vi "nanostage-reset.vi"(3 "error in":errorcluster, 4 "reset stage":bool, 5 "All conn. axes":string[](array[string])) -> (0 "error out":errorcluster, 2 "Error Description":string)   [LabVIEW 2017]
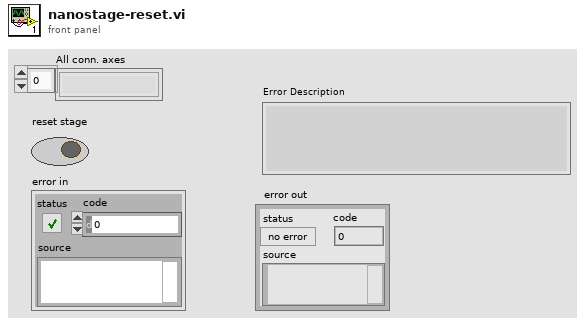
[diagram p1: front panel]
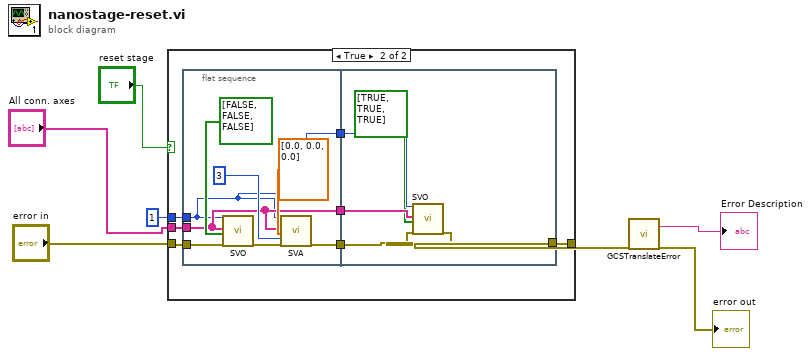
[diagram p0: block diagram]
diagram:
  n1 = case shown="True" "reset stage" {
    tunnel: "error in" -> [w8 w15]
    tunnel: [w8 w11] -> w6
    tunnel: 1 ("system no.") -> [_ w14]
    tunnel: "All conn. axes" -> [_ w13]
    frame False {
    }
    frame True {
      n2 = flat-sequence {
        tunnel: w15 -> [w23]
        tunnel: w14 -> [w16]
        tunnel: w13 -> [w17]
        tunnel: [w21] -> w12
        tunnel: [w17] -> w10
        tunnel: [w16] -> w9
        tunnel: w12 -> [w28]
        tunnel: [w27] -> w11
        tunnel: w10 -> [w26]
        tunnel: w9 -> [w25]
        frame #0 {
          n3 = call "SVO.vi"("System no."=w16, "Axes to command"=w17, "Servo mode"=bool[] [FALSE, FALSE, FALSE], "error in"=w23) -> ("error out"=w22:errorcluster)  [unwired: 15 in]
          n4 = call "SVA.vi"("System no."=w16, "Axes to move"=w17, "PZT voltage"=dbl[] [0.0, 0.0, 0.0], "No.of digits"=i16 3, "error in"=w22) -> ("error out"=w21:errorcluster)  [unwired: 14 in]
        }
        frame #1 {
          n5 = call "SVO.vi"("System no."=w25, "Axes to command"=w26, "Servo mode"=bool[] [TRUE, TRUE, TRUE], "error in"=w28) -> ("error out"=w27:errorcluster)  [unwired: 15 in]
        }
      }
    }
  }
  n6 = call "GCSTranslateError.vi"("error in"=w6) -> ("Error Description"=→"Error Description":string, "error out"=→"error out":errorcluster)  [unwired: 16 in, 1 out]
